vi "System Function Call Translator If Exists VHDL.vi"(8 "Error In":errorcluster, 11 "Node Refnum":refnum<vi>) -> (0 "Error Out":errorcluster, 1 "Defines":string[](array[string]), 2 "Includes":string[](array[string])=["<Arduino.h>", "<math.h>"], 3 "Replaced Code":string="a = floor(v);")   [LabVIEW 2018]
doc: "Run Translator.vi if it's there in same directory as SubVI. If SubVI refnum not providedd it's using VI path control."
panel:
  in  "Output Datatypes":string[](array[string])=["int"]
  in  "Input Datatypes":string[](array[string])=["error", "int"]
  in  "Outputs":string[](array[string])=["a"]
  in  "Inputs":string[](array[string])=["error in", "x"]
  in  "Function Name":string="Arduino Math.lvlib:Floor"
  # "JUST FOR NOW, DEBUGGING"
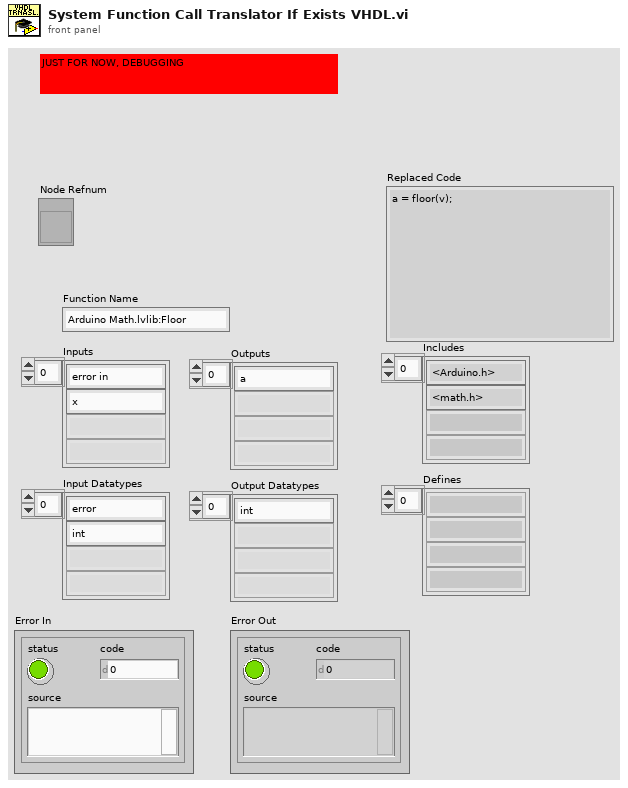
[diagram p1: front panel]
types:
  T1 = cluster{"terminals datatypes":string[][], "terminal\nconnected?":bool[], "terminal captions":string[], "term. count":i32, "terminal\nIsSource?":bool[], "SubVI name":string, "connected\nwires refs.":refnum<vi>[], "coerced dot?":bool[], "terminals[]":refnum<vi>[]}
  T2 = cluster{"wire labels":string[], "wire terminals datatypes":string[][]}
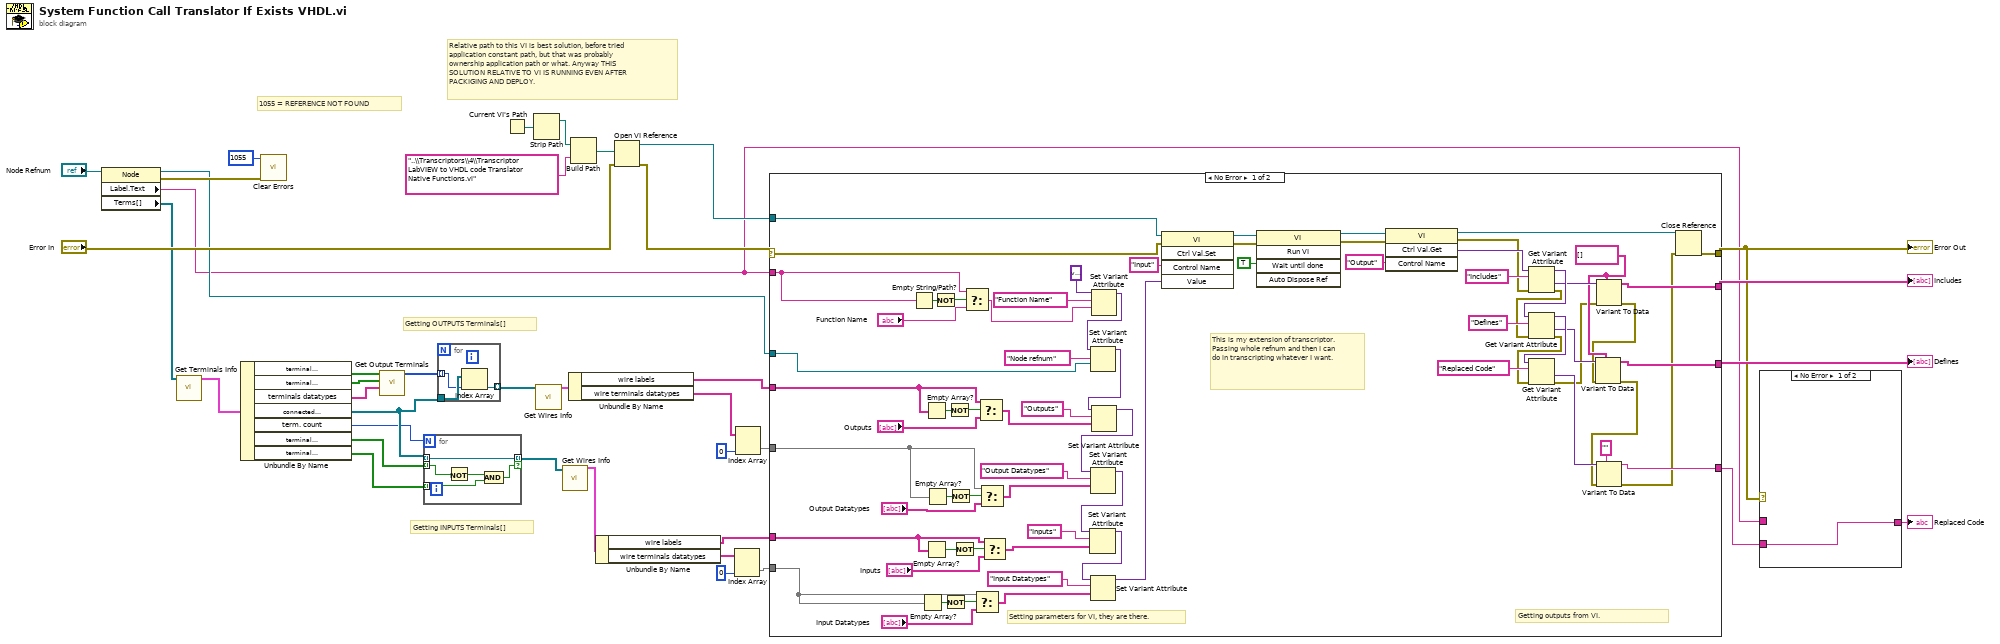
[diagram p0: block diagram]
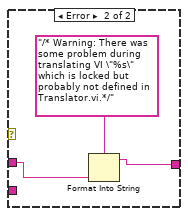
[diagram p2: hidden frame]
diagram:
  # "Relative path to this VI is best solution, before tried application constant path, but that was probably ownership application path or what. Anyway THIS SOLUTION RELATIVE TO VI IS RUNNING EVEN AFTER PACKIGING AND DEPLOY."
  # "Getting INPUTS Terminals[]"
  # "Getting OUTPUTS Terminals[]"
  # "1055 = REFERENCE NOT FOUND"
  n1 = property class="Node"(reference="Node Refnum") -> (reference out=w8:refnum<vi>, error out=w36:errorcluster, "Label.Text"=w6:string, "Terms[]"=w7:refnum<vi>[])  [unwired: 1 in]
  n2 = call "Get Terminals Info.vi"("Terms[]"=w7) -> ("output cluster"=w34:T1)  [unwired: 9 in, 1 out]
  n3 = Unbundle By Name(w34) -> ("terminal\nconnected?"=w33:bool[], "terminal\nIsSource?"=w32:bool[], "terminals datatypes"=w31:string[][], "connected\nwires refs."=w24:refnum<vi>[], "term. count"=w23:i32, "terminal\nIsSource?"=w14:bool[], "terminal\nconnected?"=w13:bool[])
  n4 = call <vilib>:"Clear Errors.vi"("error in (no error)"=w36, "specific error code to clear (0: all)"=1055) -> ()  [unwired: 4 in, 2 out]
  n5 = call "Get Output Terminals.vi"("terminals datatypes"=w31, "isSource?"=w32, "isConnected?"=w33) -> ("output terminals indexes"=w22:i32[])  [unwired: 8 in]
  n6 = for {
    N: w23 -> [_]
    tunnel: w24 -> [w43] mode=indexing
    tunnel: w14 -> [w44] mode=indexing
    tunnel: [w43] -> w12 mode=indexing if=w40
    tunnel: w13 -> [w41] mode=indexing
    n7 = Not(x=w44) -> (.not. x?=w42:bool)
    n8 = And(x=w42, y=w41) -> (x .and. y?=w40:bool)
  }
  n9 = for {
    tunnel: w22 -> [w46] mode=indexing
    tunnel: w24 -> [w47]
    tunnel: [w45] -> w30 mode=indexing
    n10 = Index Array(array=w47, index=w46) -> (element=w45:refnum<vi>)
  }
  n11 = Current VI's Path() -> (path=w3:path)
  n12 = Strip Path(path=w3) -> (stripped path=w2:path)  [unwired: 1 out]
  n13 = call "Get Wires Info.vi"("connected\nwires refs."=w30) -> ("wires info cluster"=w29:T2)  [unwired: 10 in]
  n14 = call "Get Wires Info.vi"("connected\nwires refs."=w12) -> ("wires info cluster"=w21:T2)  [unwired: 10 in]
  n15 = Unbundle By Name(w29) -> ("wire labels"=w28:string[], "wire terminals datatypes"=w27:string[][])
  n16 = Build Path(base path=w2, name or relative path="..\\Transcriptors\\4\\Transcriptor LabVIEW to VHDL code Translator Native Functions.vi") -> (appended path=w1:path)
  n17 = Unbundle By Name(w21) -> ("wire labels"=w17:string[], "wire terminals datatypes"=w19:string[][])
  n18 = Open VI Reference(vi path=w1, error in (no error)="Error In") -> (vi reference=w11:refnum<vi>, error out=w9:errorcluster)  [unwired: 4 in]
  n19 = Index Array(array=w19, index (col)=0 ("disabled index (col)")) -> (element=w18:string[])  [unwired: 1 in]
  n20 = Index Array(array=w27, index (col)=0 ("disabled index (col)")) -> (element=w25:string[])  [unwired: 1 in]
  n21 = case shown="No Error" w9 {
    selector: w9 -> [w53 w119]
    tunnel: [w118 w119] -> w16
    tunnel: [w91 _] -> w39
    tunnel: [w90 _] -> w38
    tunnel: [w89 _] -> w5
    tunnel: w28 -> [w82 _]
    tunnel: w25 -> [w69 _]
    tunnel: w18 -> [w70 _]
    tunnel: w17 -> [w62 _]
    tunnel: w11 -> [w54 _]
    tunnel: w8 -> [w49 _]
    tunnel: w6 -> [w48 _]
    frame No Error {
      w93 = string[] [] ("Array - String")
      # "This is my extension of transcriptor. Passing whole refnum and then I can do in transcripting whatever I want."
      # "Getting outputs from VI."
      # "Setting parameters for VI, they are there."
      n22 = Empty String/Path?(string/path=w48) -> (empty?=w88:bool)
      n23 = Empty Array?(array=w70) -> (empty?=w76:bool)
      n24 = Empty Array?(array=w82) -> (empty?=w81:bool)
      n25 = Empty Array?(array=w62) -> (empty?=w63:bool)
      n26 = Empty Array?(array=w69) -> (empty?=w77:bool)
      n27 = Not(x=w88) -> (.not. x?=w87:bool)
      n28 = Not(x=w76) -> (.not. x?=w75:bool)
      n29 = Not(x=w81) -> (.not. x?=w80:bool)
      n30 = Not(x=w77) -> (.not. x?=w78:bool)
      n31 = Not(x=w63) -> (.not. x?=w64:bool)
      n32 = Select(t=w48, s=w87, f="Function Name") -> (s? t:f=w86:string)
      n33 = Select(t=w70, s=w75, f="Input Datatypes") -> (s? t:f=w74:string[])
      n34 = Select(t=w82, s=w80, f="Outputs") -> (s? t:f=w79:string[])
      n35 = Select(t=w69, s=w78, f="Output Datatypes") -> (s? t:f=w73:string[])
      n36 = Select(t=w62, s=w64, f="Inputs") -> (s? t:f=w66:string[])
      n37 = Set Variant Attribute(Variant=variant ("Value"), name="Function Name", value=w86) -> (Variant out=w52:variant)  [unwired: 1 in, 2 out]
      n38 = Set Variant Attribute(Variant=w52, name="Node refnum", value=w49) -> (Variant out=w51:variant)  [unwired: 1 in, 2 out]
      n39 = Set Variant Attribute(Variant=w51, name="Outputs", value=w79) -> (Variant out=w111:variant)  [unwired: 1 in, 2 out]
      n40 = Set Variant Attribute(Variant=w111, name="Output Datatypes", value=w73) -> (Variant out=w68:variant)  [unwired: 1 in, 2 out]
      n41 = Set Variant Attribute(Variant=w68, name="Inputs", value=w66) -> (Variant out=w67:variant)  [unwired: 1 in, 2 out]
      n42 = Set Variant Attribute(Variant=w67, name="Input Datatypes", value=w74) -> (Variant out=w109:variant)  [unwired: 1 in, 2 out]
      n43 = invoke class="VI" method="Ctrl Val.Set"(reference=w54, error in=w53, "Control Name"="Input", "Value"=w109) -> (reference out=w105:refnum<vi>, error out=w104:errorcluster)  [unwired: 1 in, 3 out]
      n44 = invoke class="VI" method="Run VI"(reference=w105, error in=w104, "Wait until done"=TRUE ("Wait Until Done")) -> (reference out=w108:refnum<vi>, error out=w107:errorcluster)  [unwired: 2 in, 3 out]
      n45 = invoke class="VI" method="Ctrl Val.Get"(reference=w108, error in=w107, "Control Name"="Output") -> (reference out=w102:refnum<vi>, error out=w61:errorcluster, "Get Control Value Variant"=w103:variant)  [unwired: 1 in, 1 out]
      n46 = Get Variant Attribute(Variant=w103, name="Includes", error in=w61) -> (duplicate Variant=w98:variant, value=w96:variant, error out=w60:errorcluster)  [unwired: 1 in, 1 out]
      n47 = Get Variant Attribute(Variant=w98, name="Defines", error in=w60) -> (duplicate Variant=w97:variant, value=w95:variant, error out=w59:errorcluster)  [unwired: 1 in, 1 out]
      n48 = Get Variant Attribute(Variant=w97, name="Replaced Code", error in=w59) -> (value=w94:variant, error out=w58:errorcluster)  [unwired: 1 in, 2 out]
      n49 = Variant To Data(error in=w58, type=w93, Variant=w96) -> (data=w91:string[], error out=w57:errorcluster)
      n50 = Variant To Data(error in=w57, type=w93, Variant=w95) -> (data=w90:string[], error out=w56:errorcluster)
      n51 = Variant To Data(error in=w56, type="" ("name"), Variant=w94) -> (data=w89:string, error out=w55:errorcluster)
      n52 = Close Reference(reference=w102, error in (no error)=w55) -> (error out=w118:errorcluster)
    }
    frame Error {
    }
  }
  "Error Out" <- w16
  "Includes" <- w39
  "Defines" <- w38
  n53 = case shown="No Error" w16 {
    tunnel: [w120 w122] -> w15
    tunnel: w6 -> [_ w121]
    tunnel: w5 -> [w120 _]
    frame No Error {
    }
    frame Error {
      n54 = Format Into String(format string="/* Warning: There was some problem during translating VI \"%s\" which is locked but probably not defined in Translator.vi.*/", w121) -> (resulting string=w122:string)  [unwired: 2 in, 1 out]
    }
  }
  "Replaced Code" <- w15
